vi "TDMSFileViewer KRHPIS_edit - Copy.vi"(4 "error in (no error)":errorcluster, 7 "file path":path) -> (0 "error out":errorcluster, 3 "file path out":path)   [LabVIEW 2015]
doc: "Opens the .tdms file specified in the <B>file path</B> input and presents the file data in the TDMS File Viewer dialog box."
uses:
  <vilib>/Utility/tdmsutil.llb/fileViewerConfigData.ctl
  <vilib>/Utility/error.llb/DialogType.ctl
  <vilib>/Utility/tdmsutil.llb/TDMSFileViewerLocalizedText.vi
  Instance           1 26Saved   TDMS - File Viewer .vi
  <vilib>/Utility/file.llb/Read From Spreadsheet File (DBL).vi
  <vilib>/Analysis/NI_AALPro.lvlib
  <vilib>/Analysis/NI_AALBase.lvlib
panel:
  in  "Help":bool
  in  "Settings...":bool
  in  "Quit":bool
  in  "Status":string
  in  "Properties / Values / Graph":T1(tab)
  in  "Properties":i32(listbox)
  in  "Raw data values":i32(listbox)
  out "Time Difference 2":dbl format="%#_6p"
  out "Amplitude Difference 2":dbl format="%#_6p"
  out "Histogram":T2(graph)
  out "Waveform Graph":waveform(dbl)[](graph)
  out "St. Deviation Qin_1":dbl format="%#.4p"
  out "Variance Qin_1":dbl format="%#.4p"
  out "Mean Qin_1":dbl format="%#.4p"
  out "Mean Qin_2":dbl format="%#.4p"
  out "St. Deviation Qin_2":dbl format="%#.4p"
  out "Variance Qin_2":dbl format="%#.4p"
  out "Gain (mV/fCb)":dbl
  out "Linearity Graph":cluster{"Best Linear Fit":dbl[], "Y":dbl[]}[](graph)
  out "Pulser Waveform":waveform(dbl)[](graph)
  out "Qin 1 (fCb)":dbl format="%#.4p"
  out "Qin 2 (fCb)":dbl format="%#.4p"
  out "Simul. Graph":cluster{"all rows":dbl[], "all rows":dbl[]}[](graph)
  in  "Load simulation Plot":bool
  in  "Cursor.Visible":bool
  in  "Cursor.Visible 2":bool
  out "Time Difference":dbl format="%#_6p"
  out "Amplitude Difference":dbl format="%#_6p"
  in  "File contents":string(tree)
  # "Displaying values 1..1000"
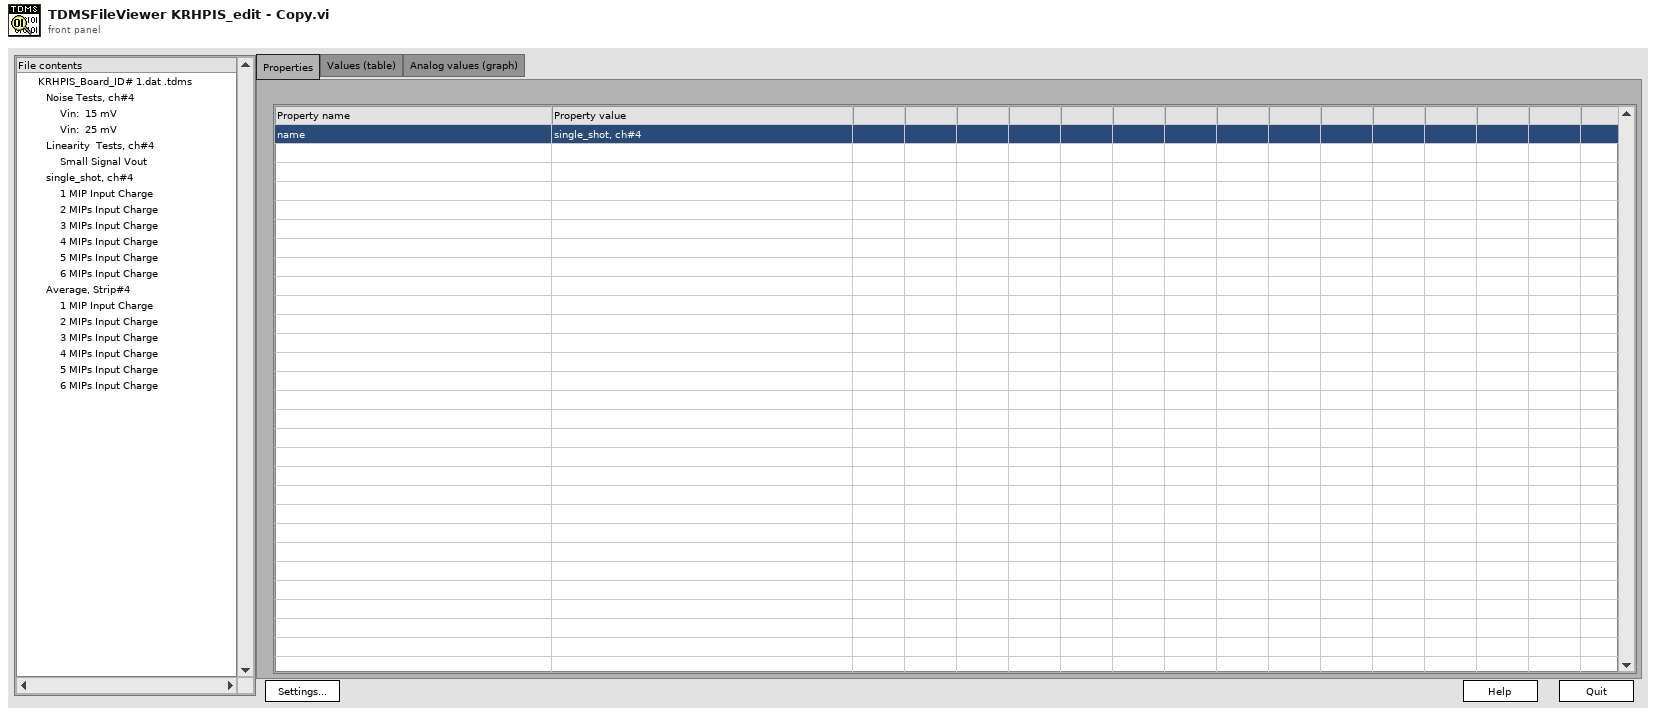
[diagram p1: front panel]
types:
  T1 = enum32{"Properties", "Values (table)", "Analog values (graph)"}
  T2 = cluster{"X Values":dbl[], "Histogram: h(x)":i32[]}[]
  T3 = enum16{"open", "open or create", "create or replace", "create", "open (read-only)"}
  T4 = typedef "fileViewerConfigData.ctl" = cluster{"Show all (table)":bool, "Show all (graph)":bool, "limit (table)":u64, "limit (graph)":u64, "no show":bool, "start (table)":u64, "start (graph)":u64}
  T5 = cluster{"Tree":refnum<vi>, "Tab Control":refnum<vi>, "property list":refnum<vi>, "raw data list":refnum<vi>, "Waveform Graph":refnum<vi>, "Ok":refnum<vi>, "Ok 2":refnum<vi>, "Ok 3":refnum<vi>, "Ok 4":refnum<vi>}
  T6 = cluster{"X Values":dbl[], "Histogram: h(x)":i32[]}
  T7 = typedef "DialogType.ctl" = u16
  T8 = typedef "LVRectTypeDef.ctl" = cluster{"Left":i16, "Top":i16, "Right":i16, "Bottom":i16}
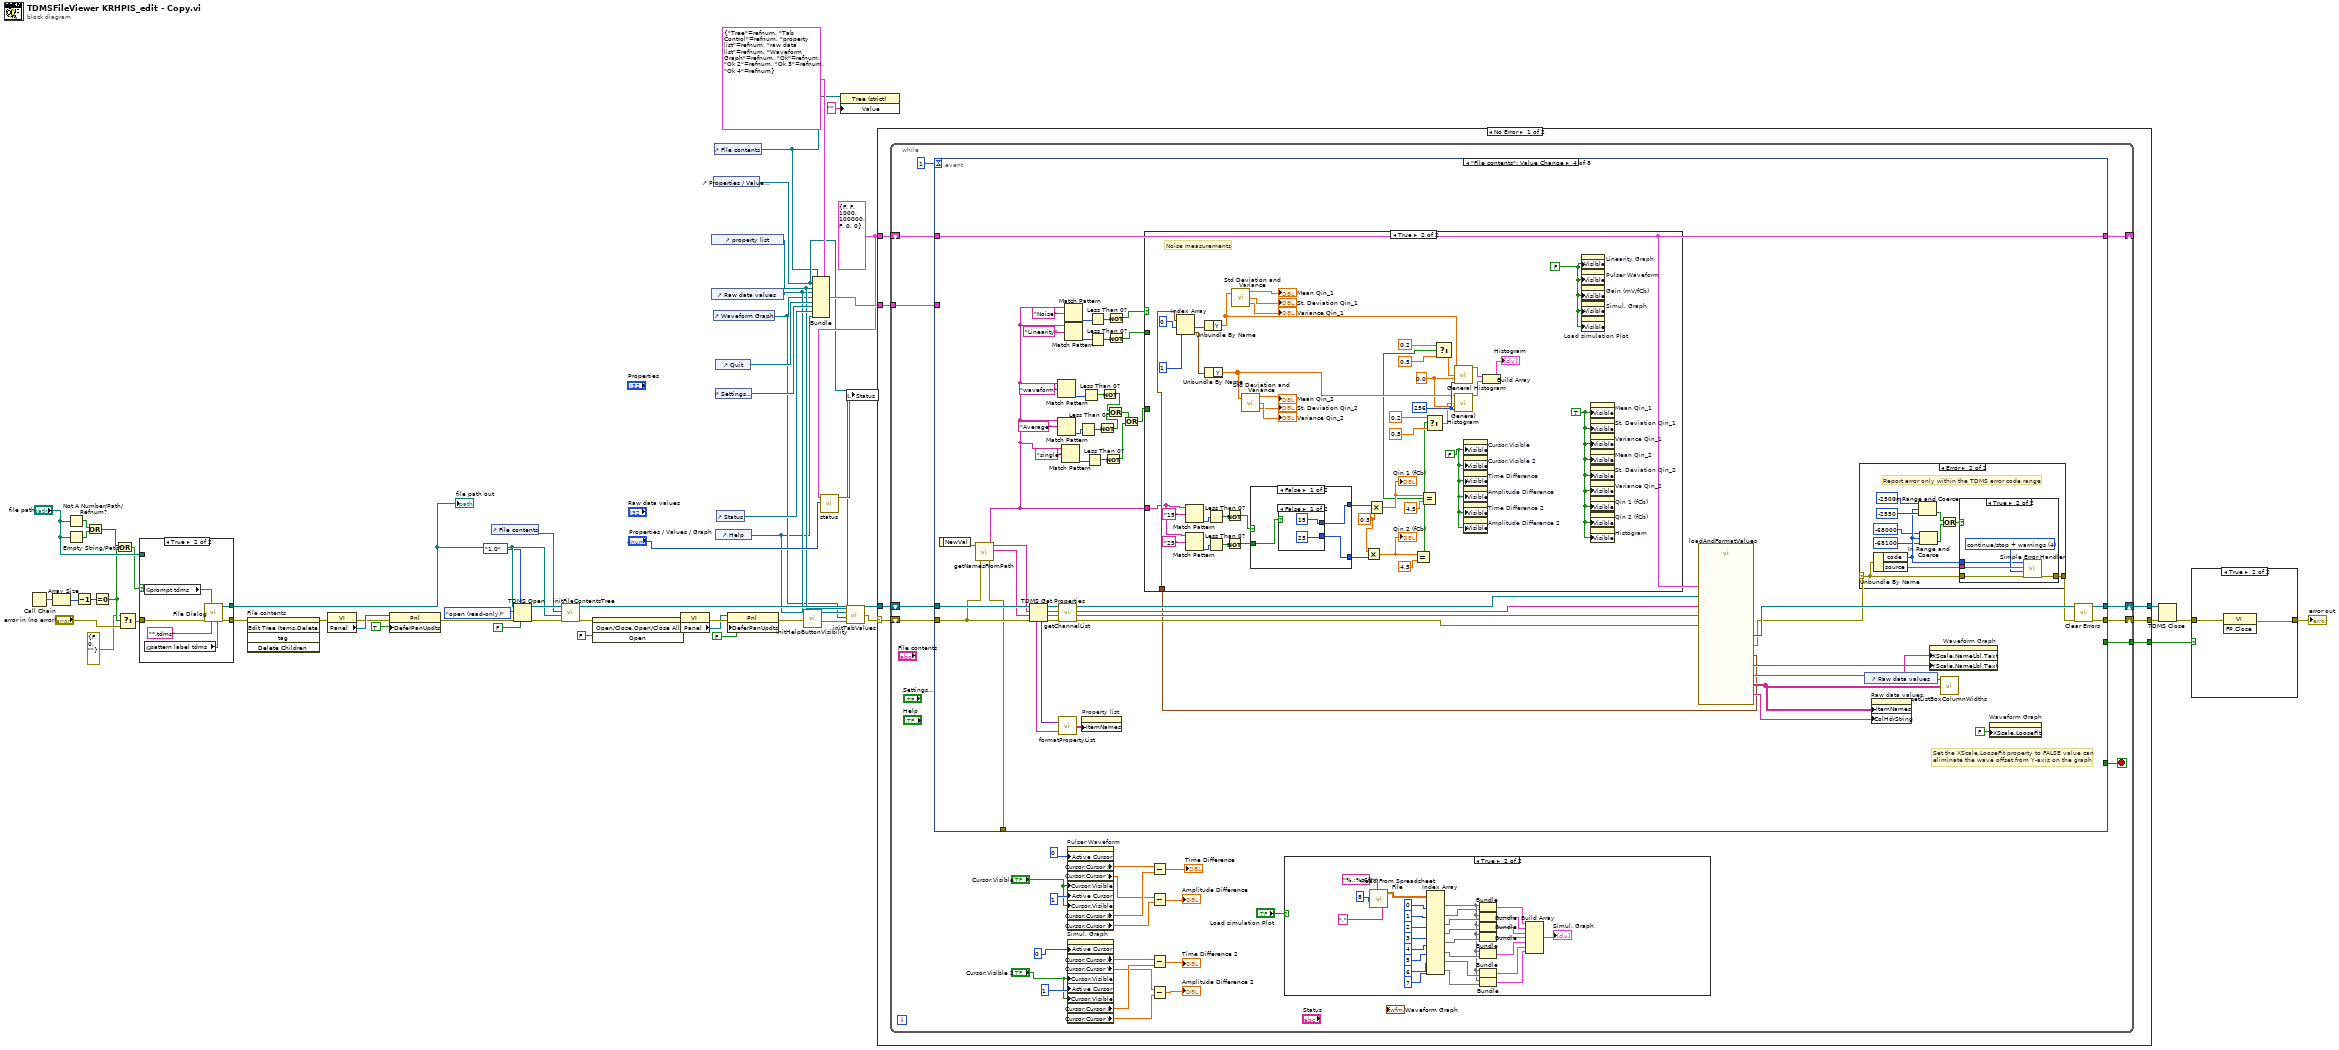
[diagram p0: block diagram]
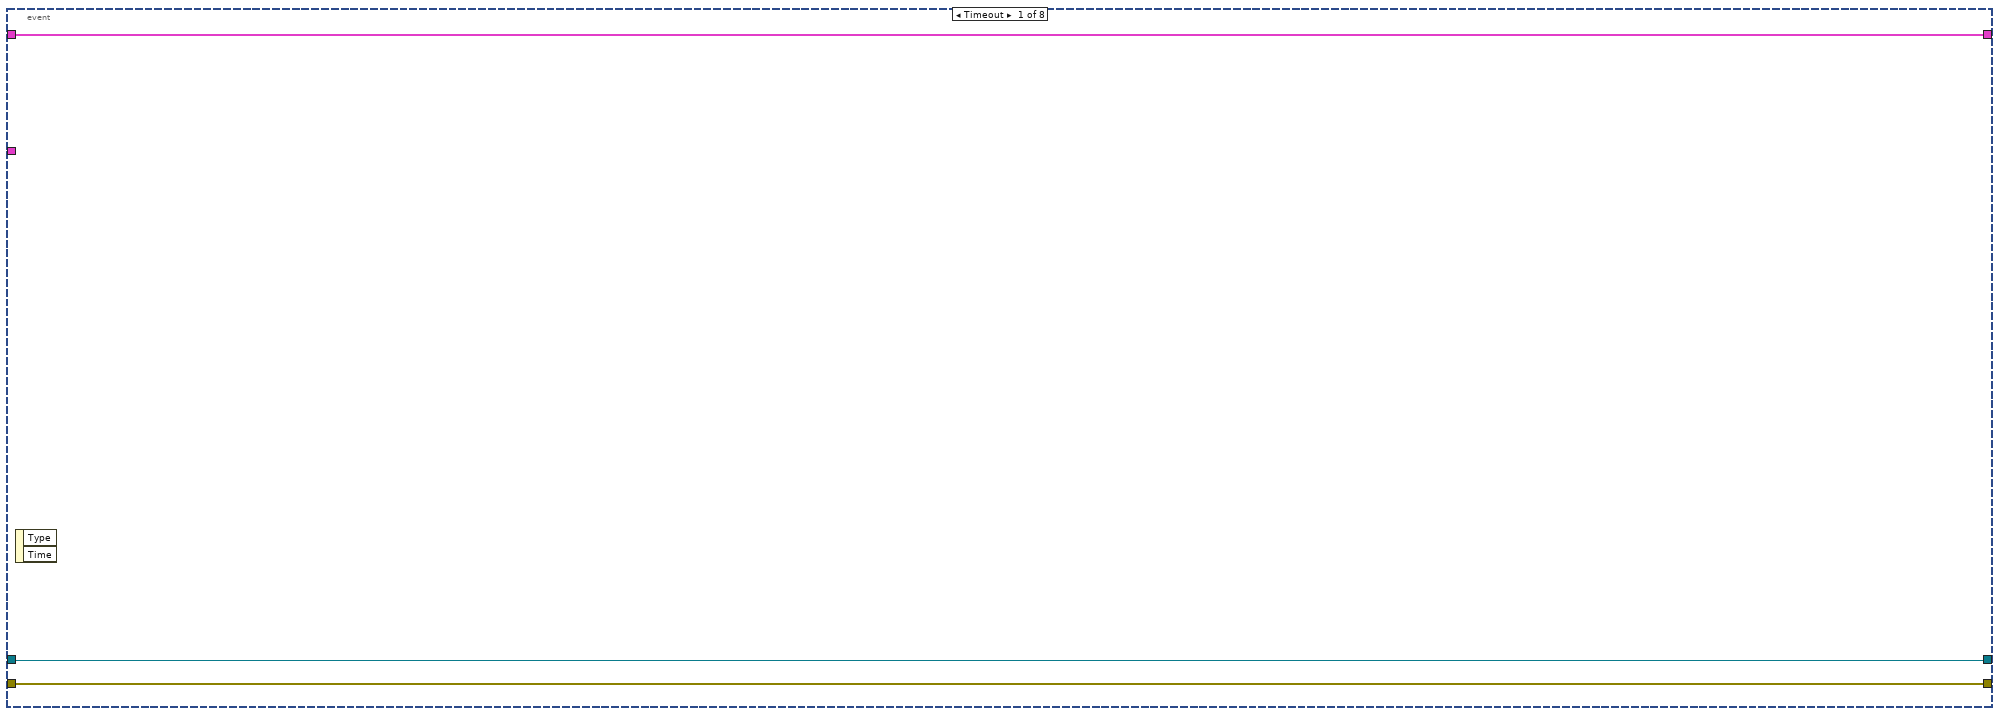
[diagram p4: hidden frame]
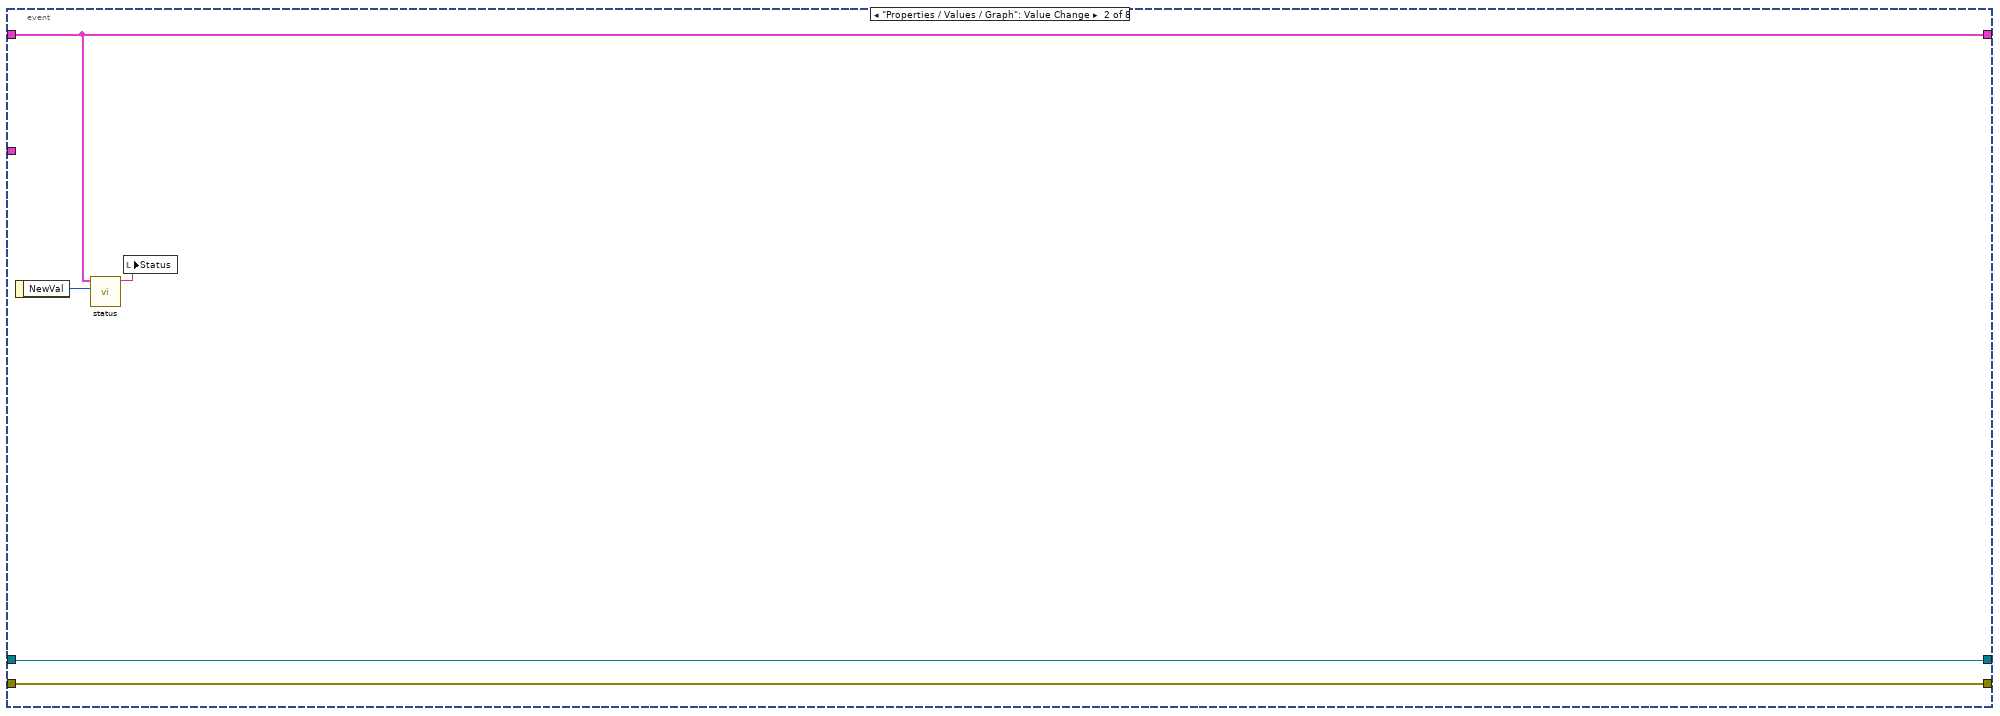
[diagram p5: hidden frame]
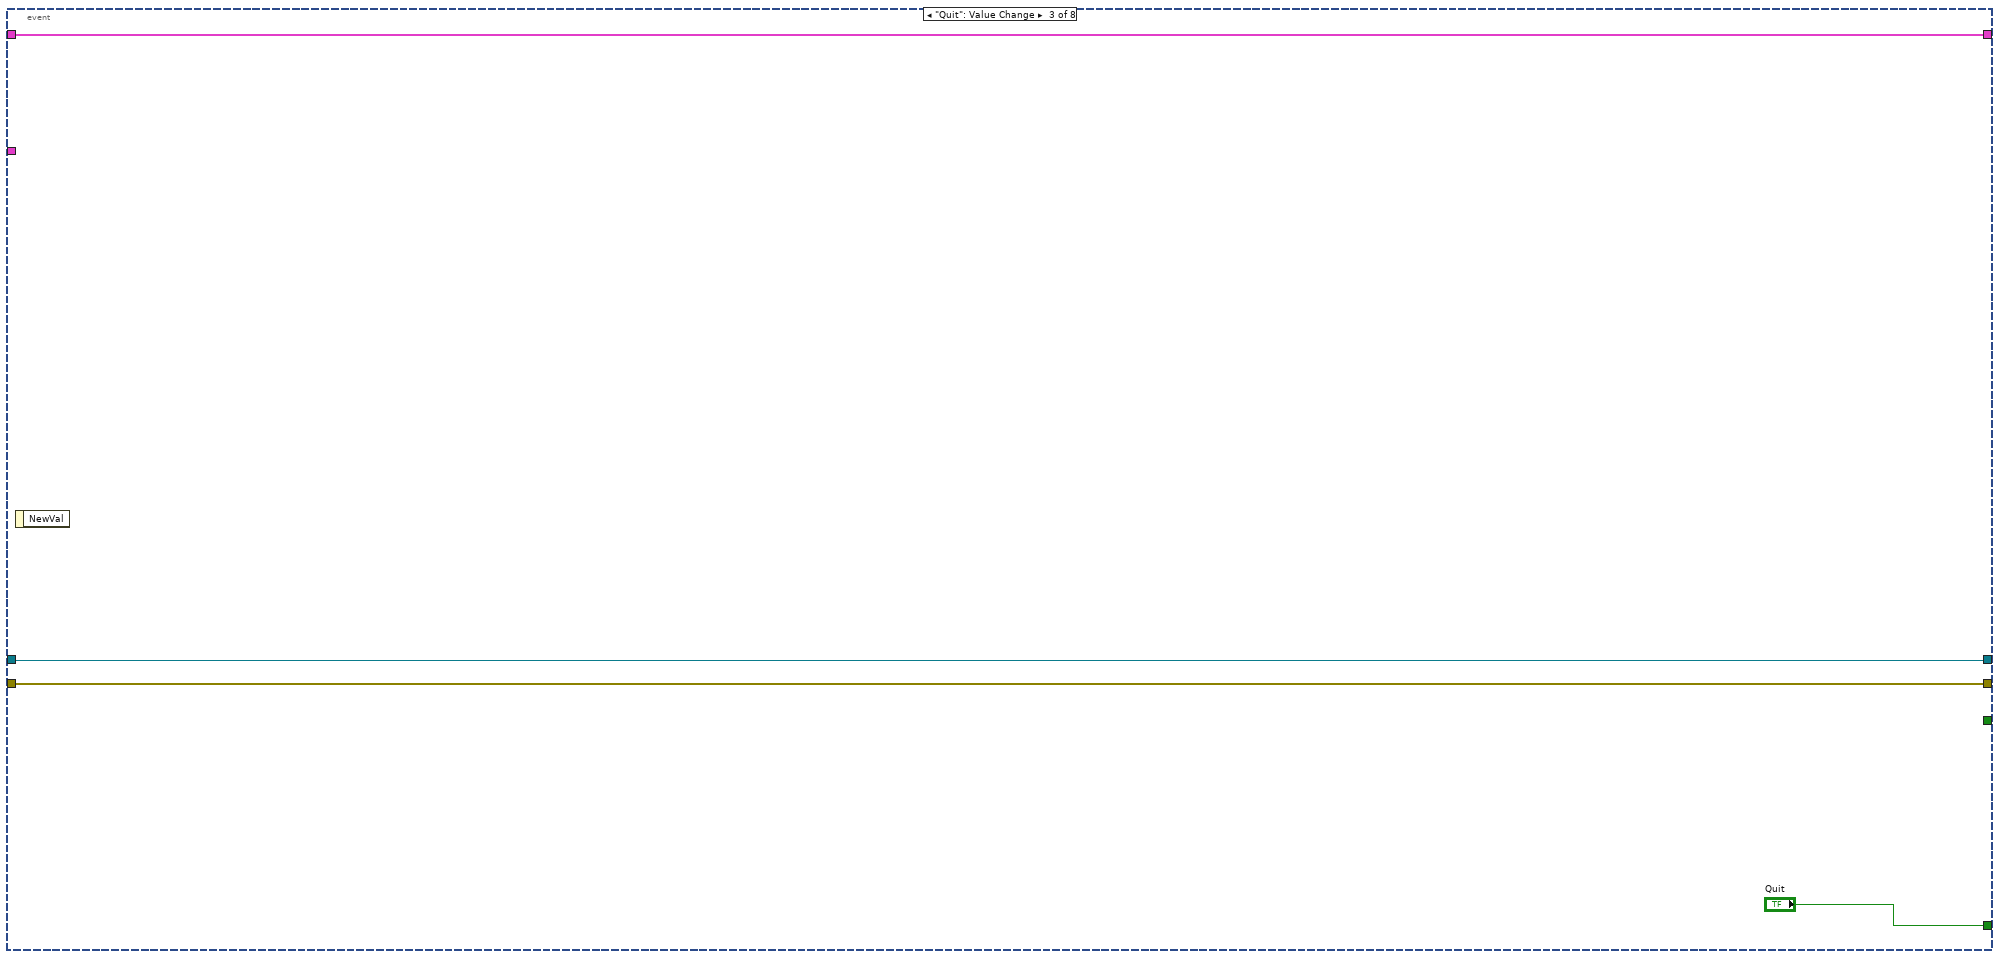
[diagram p6: hidden frame]
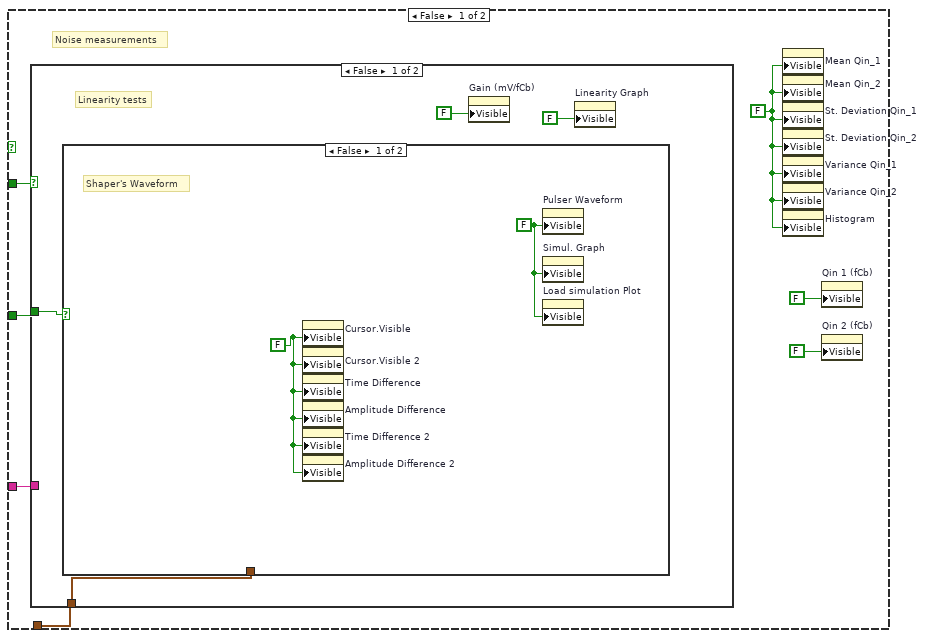
[diagram p7: hidden frame]
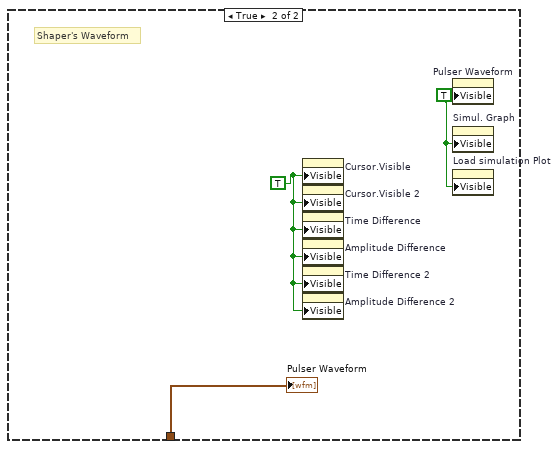
[diagram p8: hidden frame]
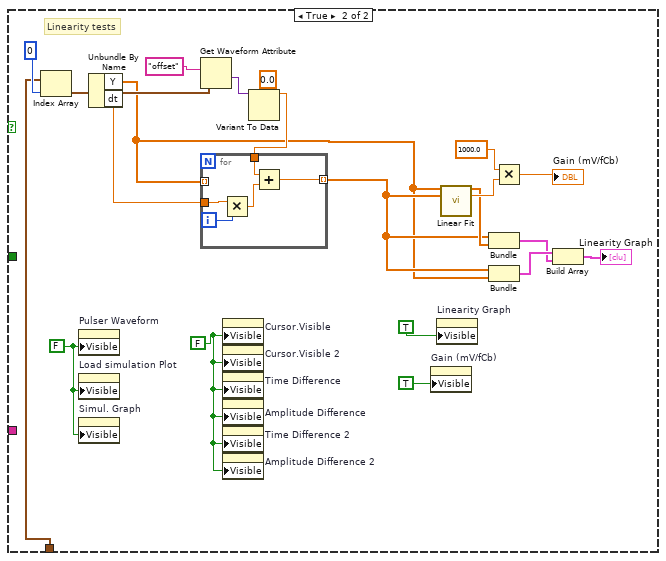
[diagram p9: hidden frame]
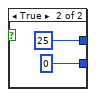
[diagram p10: hidden frame]
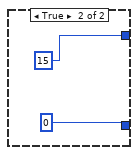
[diagram p11: hidden frame]
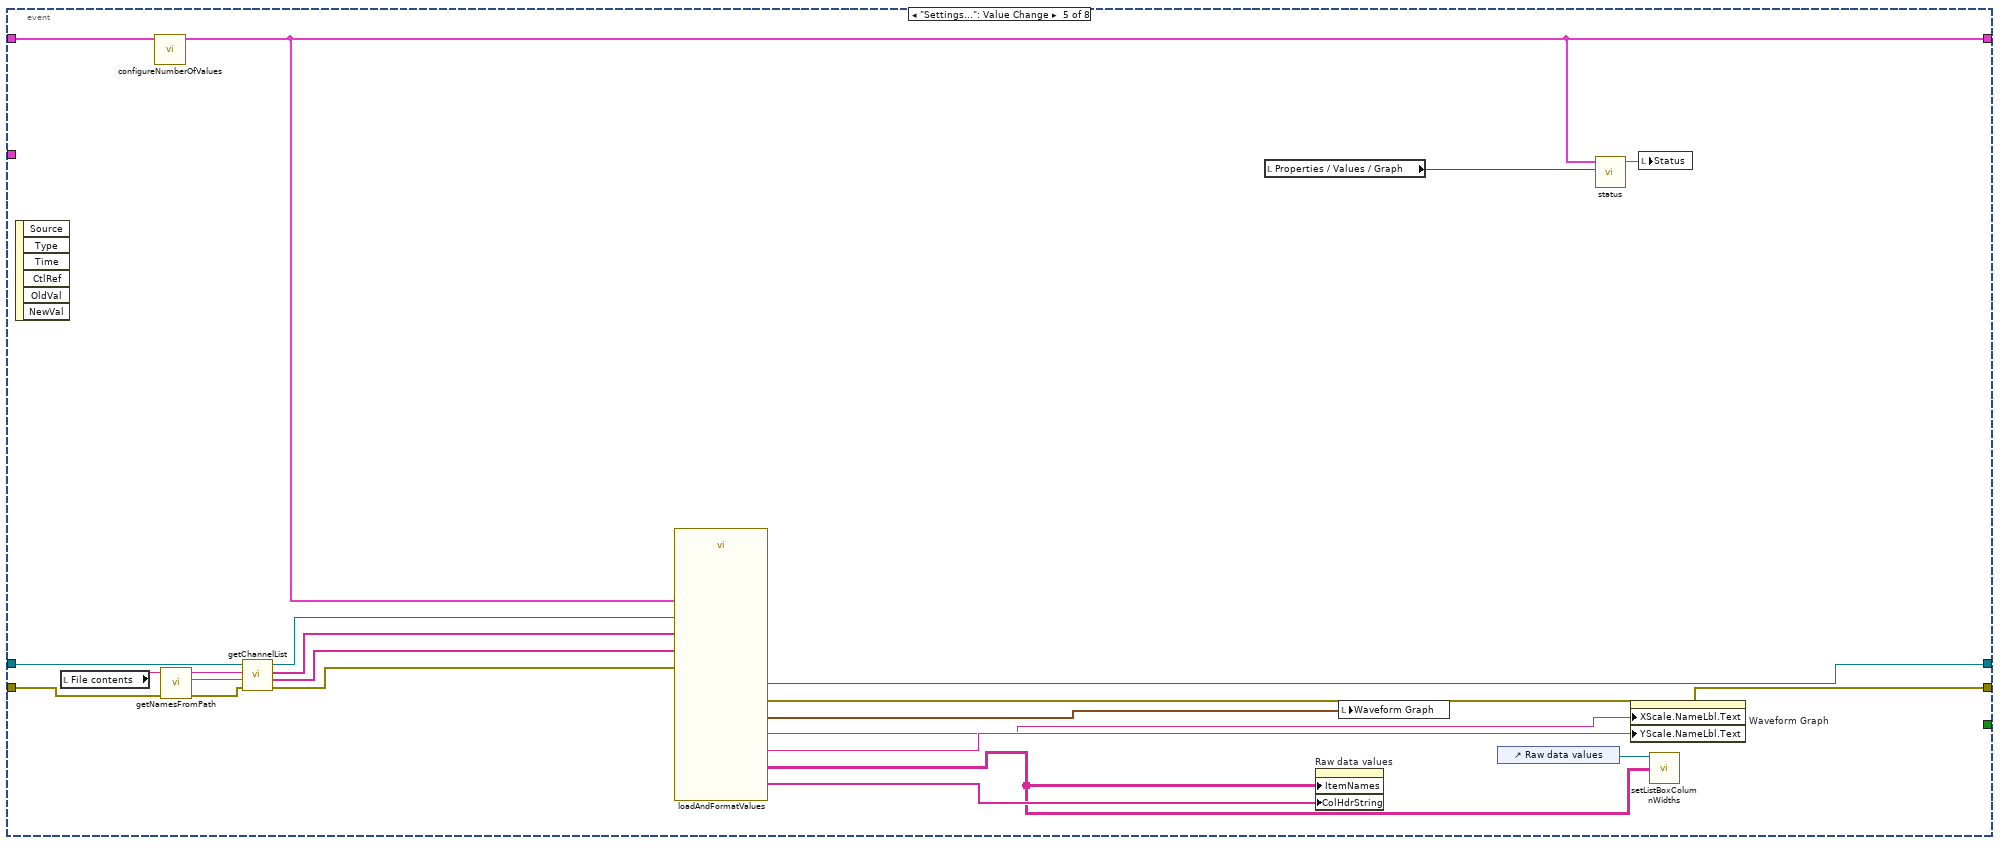
[diagram p14: hidden frame]
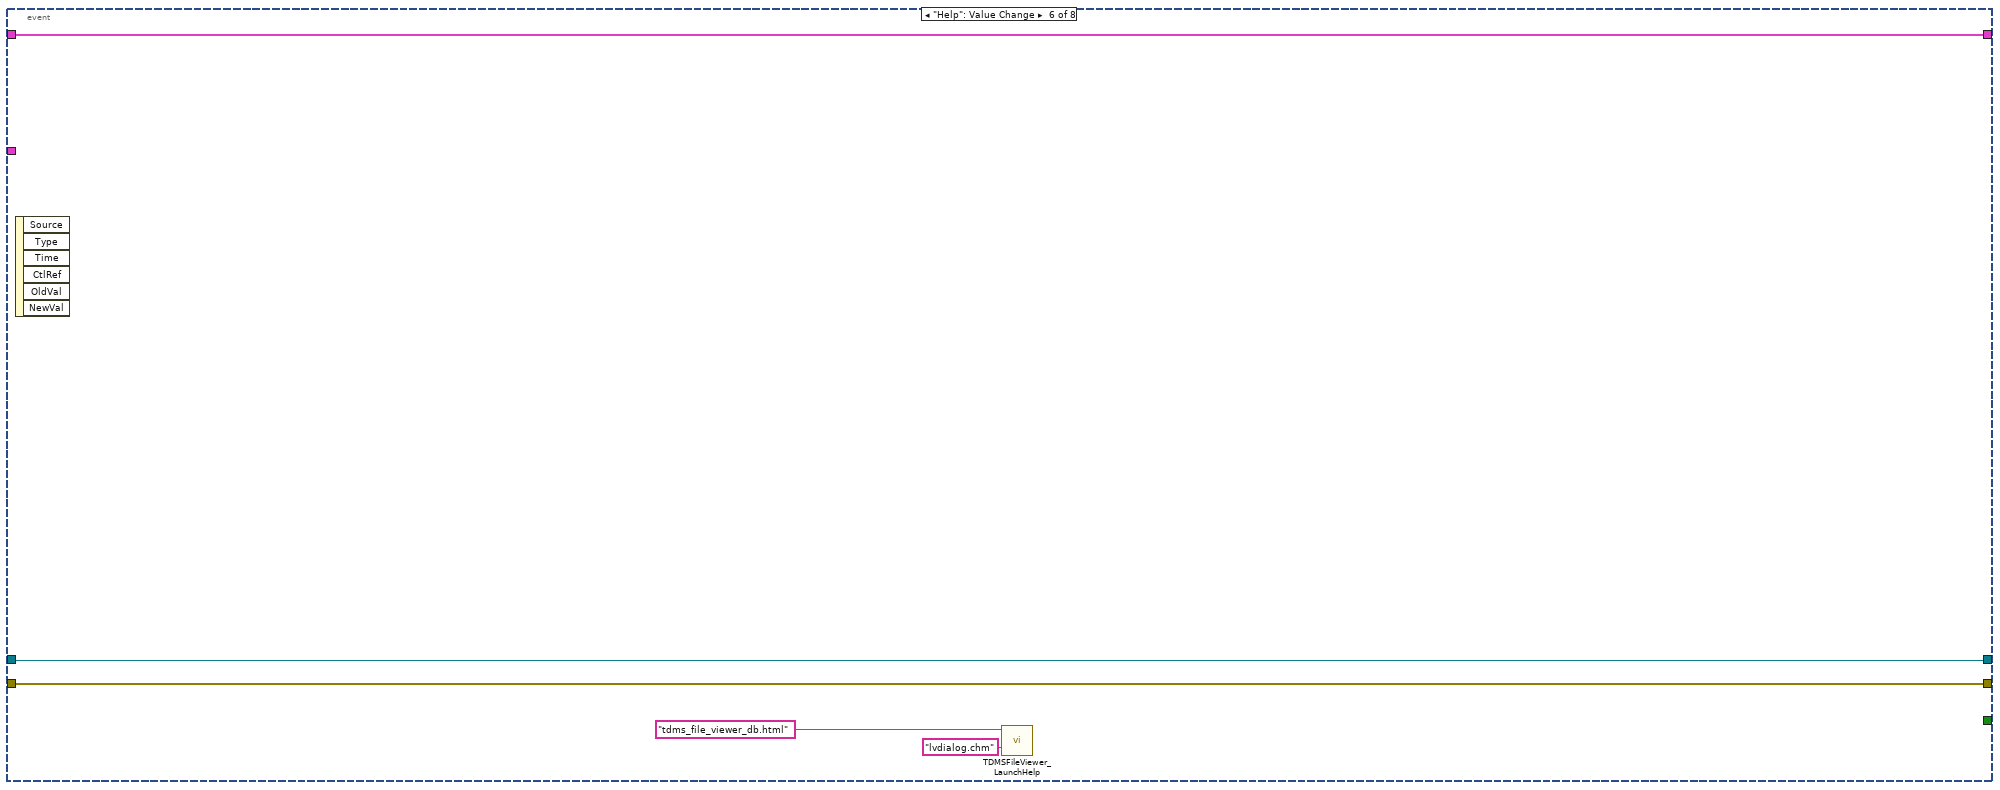
[diagram p15: hidden frame]
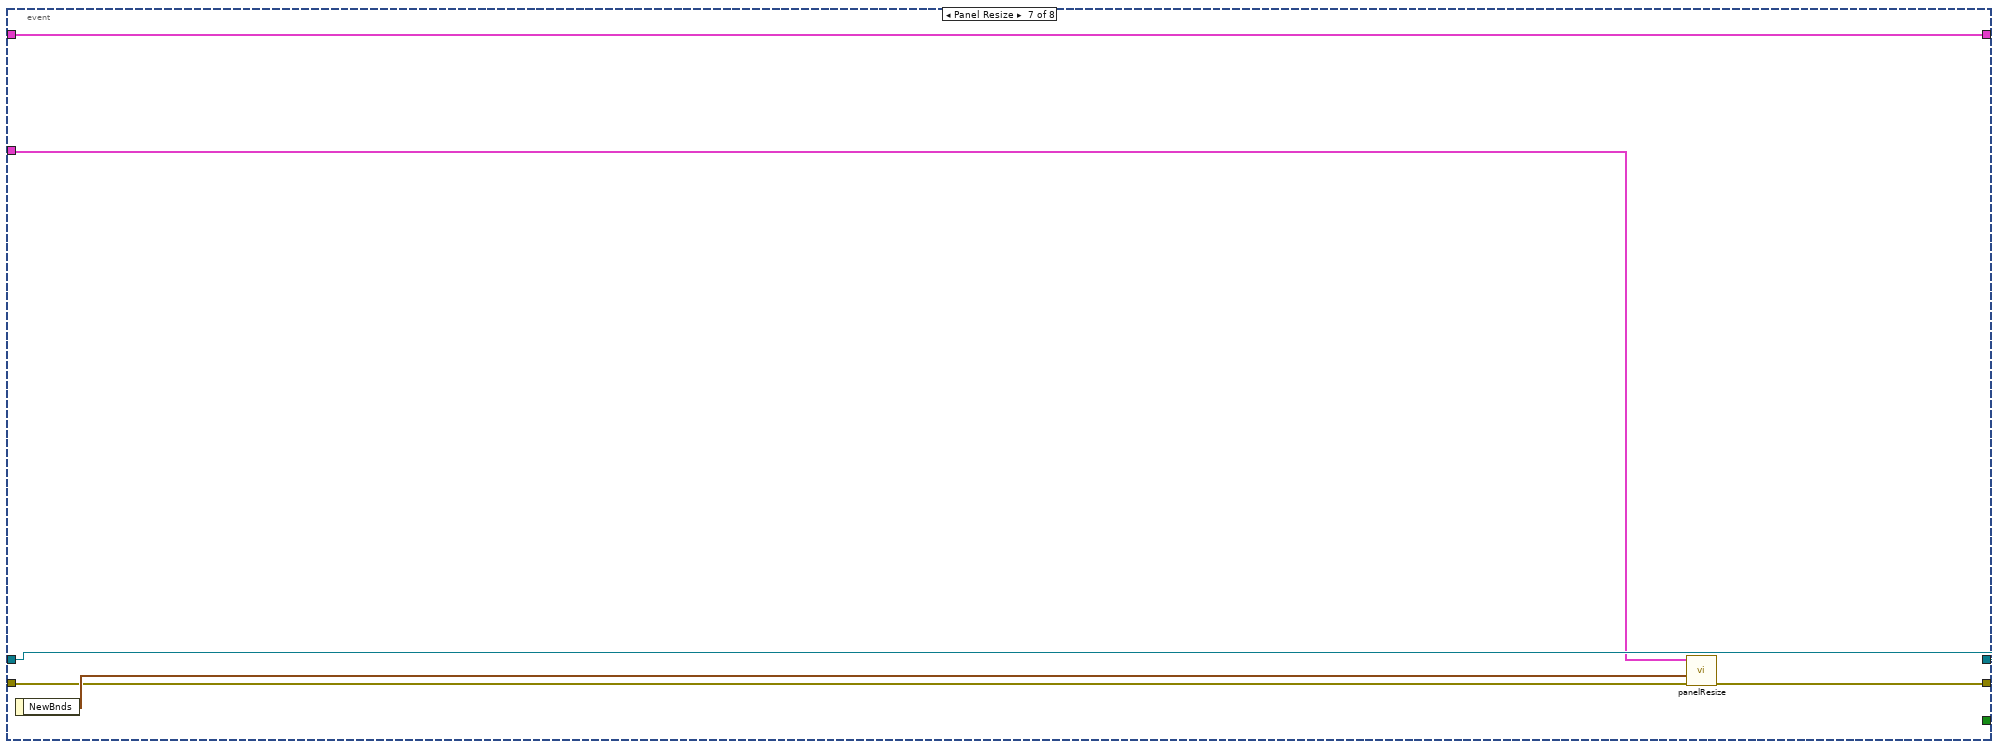
[diagram p16: hidden frame]
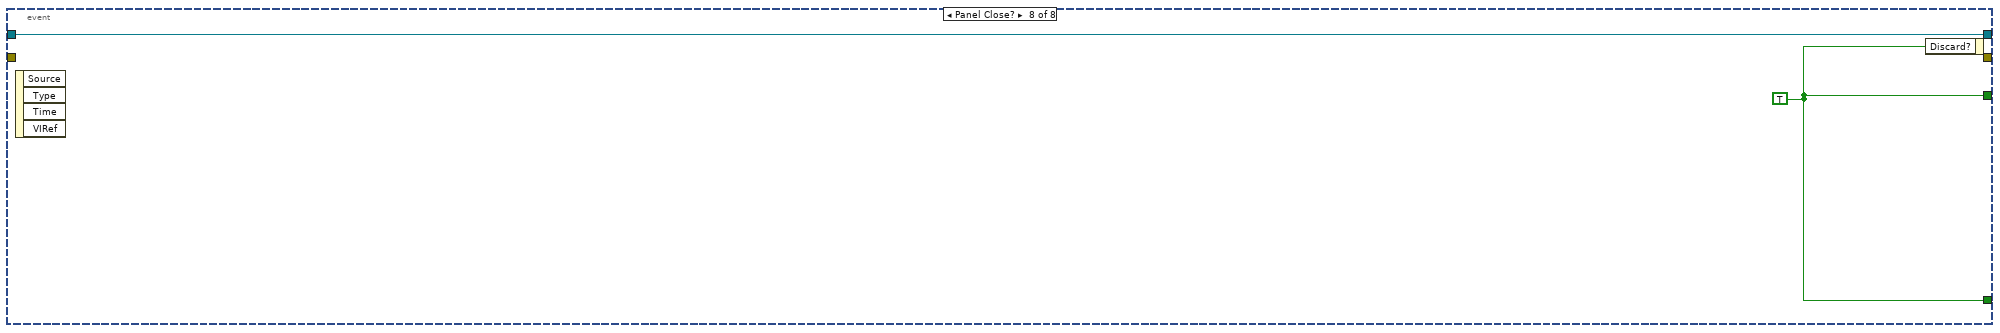
[diagram p17: hidden frame]
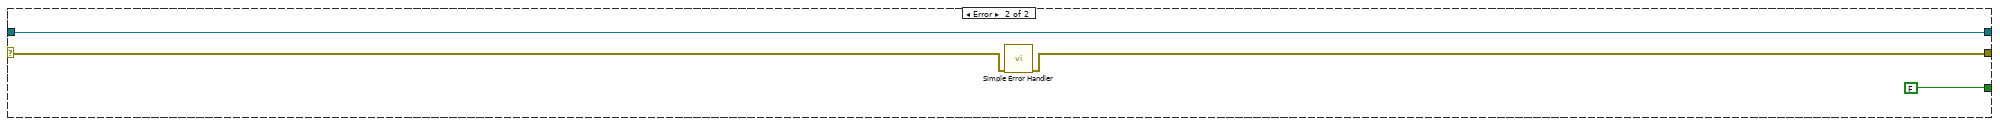
[diagram p18: hidden frame]
diagram:
  w21 = T4 {"Show all (table)"=FALSE, "Show all (graph)"=FALSE, "limit (table)"=1000, "limit (graph)"=100000, "no show"=FALSE, "start (table)"=0, "start (graph)"=0} ("TDMS File Viewer Configuration")
  n1 = Call Chain() -> (call chain=w36:string[])
  n2 = Array Size(array=w36) -> (size(s)=w34:i32)
  n3 = Not A Number/Path/Refnum?(number/path/refnum="file path") -> (NaN/Path/Refnum?=w38:bool)
  n4 = Empty String/Path?(string/path="file path") -> (empty?=w37:bool)
  n5 = Decrement(x=w34) -> (x-1=w33:i32)
  n6 = Or(x=w38, y=w37) -> (x .or. y?=w35:bool)
  n7 = Equal To 0?(x=w33) -> (x = 0?=w19:bool)
  n8 = Or(x=w35, y=w19) -> (x .or. y?=w32:bool)
  n9 = Select(t=errorcluster {"status"=FALSE, "code"=0, "source"=""}, s=w19, f="error in (no error)") -> (s? t:f=w18:errorcluster)
  n10 = case shown="True" w32 {
    tunnel: [w57 w63] -> w25
    tunnel: "file path" -> [w57 _]
    tunnel: [w56 w61] -> w24
    tunnel: w18 -> [w56 w60]
    frame False {
    }
    frame True {
      n11 = global read "TDMSFileViewerLocalizedText.vi" "prompt tdms"() -> (w59:string)
      n12 = global read "TDMSFileViewerLocalizedText.vi" "pattern label tdms"() -> (w58:string)
      n13 = call "File Dialog"("prompt"=w59, "error in"=w60, "pattern (all files)"="*.tdms", "pattern label"=w58) -> ("selected path"=w63:path, "error out"=w61:errorcluster)  [unwired: 3 in, 7 out]
    }
  }
  "file path out" <- w25
  n14 = invoke on="File contents" class="Tree (strict)" method="Edit Tree Items.Delete"(error in=w24) -> (error out=w46:errorcluster)  [unwired: 4 in, 4 out]
  n15 = property class="VI"(error in=w46) -> (error out=w47:errorcluster, "Panel"=w48:refnum<vi>)  [unwired: 1 in, 1 out]
  n16 = property class="Pnl"(reference=w48, error in=w47, "DeferPanUpdts"=TRUE ("Defer Panel Updates")) -> (error out=w50:errorcluster)  [unwired: 1 out]
  n17 = control-ref of="File contents"() -> (w26:refnum<vi>)
  n18 = TDMS Open(6:FALSE ("disable buffering (T)"), 7:enum16{"1.0", "2.0"}."1.0" ("file format version (2.0)"), 8:w50, 10:T3."open (read-only)" ("operation"), 11:w25) -> (0:w55:errorcluster, 3:w54:refnum<k34>)  [unwired: 2 in]
  n19 = call <vilib>:"initFileContentsTree.vi"("error in (no error)"=w55, "file path"=w25, "Tree Refnum"=w26, "tdms file"=w54) -> ("error out"=w42:errorcluster, "tdms file out"=w53:refnum<k34>)  [unwired: 2 out]
  n20 = invoke on="File contents" class="Tree (strict)" method="Open/Close.Open/Close All"(error in=w42, "Open"=FALSE ("Open?")) -> (error out=w41:errorcluster)  [unwired: 2 in, 3 out]
  n21 = property class="VI"(error in=w41) -> (error out=w44:errorcluster, "Panel"=w43:refnum<vi>)  [unwired: 1 in, 1 out]
  n22 = control-ref of="property list"() -> (w9:refnum<vi>)
  n23 = control-ref of="Raw data values"() -> (w8:refnum<vi>)
  n24 = control-ref of="Properties / Values / Graph"() -> (w6:refnum<vi>)
  n25 = control-ref of="Waveform Graph"() -> (w7:refnum<vi>)
  n26 = control-ref of="File contents"() -> (w5:refnum<vi>)
  n27 = control-ref of="Quit"() -> (w30:refnum<vi>)
  n28 = control-ref of="Settings..."() -> (w28:refnum<vi>)
  n29 = control-ref of="Help"() -> (w1:refnum<vi>)
  n30 = control-ref of="Status"() -> (w23:refnum<vi>)
  n31 = property class="Pnl"(reference=w43, error in=w44, "DeferPanUpdts"=FALSE ("Defer Panel Updates")) -> (error out=w3:errorcluster)  [unwired: 1 out]
  n32 = call <vilib>:"initHelpButtonVisibility.vi"("error in"=w3, "Help"=w1) -> ("error out"=w2:errorcluster)  [unwired: 9 in]
  n33 = Bundle(cluster=T5 {"Tree"=refnum, "Tab Control"=refnum, "property list"=refnum, "raw data list"=refnum, "Waveform Graph"=refnum, "Ok"=refnum, "Ok 2"=refnum, "Ok 3"=refnum, "Ok 4"=refnum} ("control refs"), "Tree"=w5, "Tab Control"=w6, "property list"=w9, "raw data list"=w8, "Waveform Graph"=w7, "Ok"=w30, "Ok 2"=w28, "Ok 3"=w23, "Ok 4"=w1) -> (w31:T5)
  n34 = call <vilib>:"status.vi"("tab sheet"="Properties / Values / Graph", "TDMS File Viewer Configuration"=w21) -> ("status"=w22:string)  [unwired: 5 out]
  n35 = property class="Tree (strict)"(reference=w5, "Value"="") -> ()  [unwired: 1 in, 2 out]
  n36 = local write "Status"(w22) -> ()
  n37 = call <vilib>:"initTabValues.vi"("properties"=w9, "Values"=w8, "waveform"=w7, "error in"=w2, "Properties / Values / Graph"=w6) -> ("error out"=w10:errorcluster)
  n38 = case shown="No Error" w10 {
    selector: w10 -> [w65 w342]
    tunnel: w53 -> [w70 w343]
    tunnel: [w69 w343] -> w52
    tunnel: [w68 w341] -> w51
    tunnel: w31 -> [w67 _]
    tunnel: w21 -> [w66 _]
    tunnel: [w64 FALSE] -> w15
    frame No Error {
      n39 = while {
        shift-right: [w97] -> w68
        shift-left: w65 -> [w98]
        shift-right: [w96] -> w69
        shift-left: w70 -> [w99]
        tunnel: w67 -> [w94]
        shift-right: [w92] -> _
        shift-left: w66 -> [w93]
        tunnel: [w91] -> w64
        stop <- w95 stop-if-true
        n40 = event shown="[3] \"File contents\": Value Change" {
          selector: _ -> [_ _ _ _ _ _ _ _]
          dyn-events: _ -> [_ _ _ _ _ _ _ _]
          timeout: 1 -> [_ _ _ _ _ _ _ _]
          tunnel: w99 -> [w129 w134 w138 w190 w315 w330 w337 w339]
          tunnel: w98 -> [w130 w135 w137 w183 w323 w329 w334 _]
          tunnel: [w130 w135 w137 w179 w324 w329 w333 _] -> w97
          tunnel: [w129 w134 w138 w189 w325 w330 w337 w339] -> w96
          tunnel: [_ _ "Quit" _ _ _ _ w338] -> w95
          tunnel: [_ _ _ w182 _ _ _ _] -> _
          tunnel: w94 -> [_ _ _ _ _ _ w335 _]
          tunnel: w93 -> [w128 w131 w136 w172 w326 w331 w332 _]
          tunnel: [w128 w131 w136 w172 w305 w331 w332 _] -> w92
          tunnel: [_ _ _ _ _ _ _ w338] -> w91
          event Timeout {
            n41 = event-data() -> ()  [unwired: 3 out]
          }
          event "Properties / Values / Graph": Value Change {
            n42 = event-data() -> ("NewVal"=w133:T1)  [unwired: 1 out]
            n43 = call <vilib>:"status.vi"("tab sheet"=w133, "TDMS File Viewer Configuration"=w131) -> ("status"=w132:string)  [unwired: 5 out]
            n44 = local write "Status"(w132) -> ()
          }
          event "Quit": Value Change {
            n45 = event-data() -> ()  [unwired: 2 out]
          }
          event "File contents": Value Change {
            # "Set the XScale.LooseFit property to FALSE value can \neliminate the wave offset from Y-axis on the graph"
            n46 = event-data() -> ("NewVal"=w143:string)  [unwired: 1 out]
            n47 = call <vilib>:"getNamesFromPath.vi"("error in (no error)"=w183, "tree path"=w143) -> ("error out"=w182:errorcluster, "channel"=w187:string, "group"=w188:string)  [unwired: 3 out]
            n48 = TDMS Get Properties(8:w183, 9:w187, 10:w188, 11:w190) -> (0:w177:errorcluster, 1:w176:string, 2:w171:string, 3:w178:refnum<k34>, 4:w185:variant[], 6:w186:string[])  [unwired: 2 out]
            n49 = Match Pattern(string=w143, regular expression="waveform") -> (offset past match=w158:i32)  [unwired: 1 in, 3 out]
            n50 = Match Pattern(string=w143, regular expression="Average") -> (offset past match=w150:i32)  [unwired: 1 in, 3 out]
            n51 = call <vilib>:"getChannelList.vi"("error in (no error)"=w177, "channel names"=w176, "group name"=w171, "tdms file"=w178) -> ("error out"=w167:errorcluster, "channel names out"=w168:string[], "group names out"=w169:string[], "tdms file out"=w170:refnum<k34>)
            n52 = call <vilib>:"formatPropertyList.vi"("property names"=w186, "property values"=w185) -> ("strings"=w184:string[][])
            n53 = Match Pattern(string=w143, regular expression="single") -> (offset past match=w145:i32)  [unwired: 1 in, 3 out]
            n54 = Match Pattern(string=w143, regular expression="Noise") -> (offset past match=w162:i32)  [unwired: 1 in, 3 out]
            n55 = Match Pattern(string=w143, regular expression="Linearity") -> (offset past match=w160:i32)  [unwired: 1 in, 3 out]
            n56 = Less Than 0?(x=w150) -> (x < 0?=w151:bool)
            n57 = property on="Property list" class="MCListbox (strict)"("ItemNames"=w184) -> ()  [unwired: 2 in, 2 out]
            n58 = Less Than 0?(x=w158) -> (x < 0?=w155:bool)
            n59 = Less Than 0?(x=w145) -> (x < 0?=w144:bool)
            n60 = Less Than 0?(x=w162) -> (x < 0?=w157:bool)
            n61 = Less Than 0?(x=w160) -> (x < 0?=w156:bool)
            n62 = Not(x=w151) -> (.not. x?=w149:bool)
            n63 = Not(x=w155) -> (.not. x?=w148:bool)
            n64 = Not(x=w144) -> (.not. x?=w142:bool)
            n65 = Or(x=w148, y=w149) -> (x .or. y?=w141:bool)
            n66 = Not(x=w157) -> (.not. x?=w154:bool)
            n67 = Not(x=w156) -> (.not. x?=w153:bool)
            n68 = Or(x=w141, y=w142) -> (x .or. y?=w140:bool)
            n69 = call <vilib>:"loadAndFormatValues.vi"("error in (no error)"=w167, "configuration"=w172, "channel names"=w168, "group names"=w169, "tdms file"=w170) -> ("error out"=w166:errorcluster, "graph y names"=w174:string, "graph x names"=w173:string, "tdms file out"=w189:refnum<k34>, "waveform values"=w147:waveform(dbl)[], "table values"=w181:string[][], "table headers"=w175:string[])
            n70 = case shown="True" w154 {
              tunnel: w147 -> [w196 w267]
              tunnel: w153 -> [w197 _]
              tunnel: w143 -> [w195 w253]
              tunnel: w140 -> [w194 _]
              frame False {
                w193 = FALSE ("Visible")
                # "Noise measurements"
                n71 = case shown="False" w197 {
                  tunnel: w196 -> [w199 w226]
                  tunnel: w195 -> [_ _]
                  tunnel: w194 -> [w201 _]
                  frame False {
                    # "Linearity tests"
                    n72 = case shown="False" w201 {
                      tunnel: w199 -> [_ w206]
                      frame False {
                        w202 = FALSE ("Cursor.Visible")
                        w203 = FALSE ("Visible")
                        # "Shaper's Waveform"
                        n73 = property on="Cursor.Visible" class="Bool (strict)"("Visible"=w202) -> ()  [unwired: 2 in, 2 out]
                        n74 = property on="Cursor.Visible 2" class="Bool (strict)"("Visible"=w202) -> ()  [unwired: 2 in, 2 out]
                        n75 = property on="Time Difference" class="DigNum (strict)"("Visible"=w202) -> ()  [unwired: 2 in, 2 out]
                        n76 = property on="Amplitude Difference" class="DigNum (strict)"("Visible"=w202) -> ()  [unwired: 2 in, 2 out]
                        n77 = property on="Time Difference 2" class="DigNum (strict)"("Visible"=w202) -> ()  [unwired: 2 in, 2 out]
                        n78 = property on="Amplitude Difference 2" class="DigNum (strict)"("Visible"=w202) -> ()  [unwired: 2 in, 2 out]
                        n79 = property on="Pulser Waveform" class="WFGraph (strict)"("Visible"=w203) -> ()  [unwired: 2 in, 2 out]
                        n80 = property on="Simul. Graph" class="XYGraph (strict)"("Visible"=w203) -> ()  [unwired: 2 in, 2 out]
                        n81 = property on="Load simulation Plot" class="Bool"("Visible"=w203) -> ()  [unwired: 2 in, 2 out]
                      }
                      frame True {
                        w204 = TRUE ("Cursor.Visible")
                        w205 = TRUE ("Visible")
                        # "Shaper's Waveform"
                        n82 = property on="Cursor.Visible" class="Bool (strict)"("Visible"=w204) -> ()  [unwired: 2 in, 2 out]
                        n83 = property on="Cursor.Visible 2" class="Bool (strict)"("Visible"=w204) -> ()  [unwired: 2 in, 2 out]
                        n84 = property on="Time Difference" class="DigNum (strict)"("Visible"=w204) -> ()  [unwired: 2 in, 2 out]
                        n85 = property on="Amplitude Difference" class="DigNum (strict)"("Visible"=w204) -> ()  [unwired: 2 in, 2 out]
                        n86 = property on="Time Difference 2" class="DigNum (strict)"("Visible"=w204) -> ()  [unwired: 2 in, 2 out]
                        n87 = property on="Amplitude Difference 2" class="DigNum (strict)"("Visible"=w204) -> ()  [unwired: 2 in, 2 out]
                        n88 = property on="Pulser Waveform" class="WFGraph (strict)"("Visible"=w205) -> ()  [unwired: 2 in, 2 out]
                        n89 = property on="Simul. Graph" class="XYGraph (strict)"("Visible"=w205) -> ()  [unwired: 2 in, 2 out]
                        n90 = property on="Load simulation Plot" class="Bool"("Visible"=w205) -> ()  [unwired: 2 in, 2 out]
                        "Pulser Waveform" <- w206
                      }
                    }
                    n91 = property on="Gain (mV/fCb)" class="DigNum (strict)"("Visible"=FALSE) -> ()  [unwired: 2 in, 2 out]
                    n92 = property on="Linearity Graph" class="XYGraph (strict)"("Visible"=FALSE) -> ()  [unwired: 2 in, 2 out]
                  }
                  frame True {
                    w216 = FALSE ("Cursor.Visible")
                    w217 = FALSE ("Visible")
                    # "Linearity tests"
                    n93 = Index Array(array=w226, index=0) -> (element=w214:waveform(dbl))
                    n94 = property on="Pulser Waveform" class="WFGraph (strict)"("Visible"=w217) -> ()  [unwired: 2 in, 2 out]
                    n95 = property on="Load simulation Plot" class="Bool"("Visible"=w217) -> ()  [unwired: 2 in, 2 out]
                    n96 = property on="Simul. Graph" class="XYGraph (strict)"("Visible"=w217) -> ()  [unwired: 2 in, 2 out]
                    n97 = Unbundle By Name(w214) -> ("Y"=w207:dbl[], "dt"=w210:dbl)
                    n98 = Get Waveform Attribute(6:"offset" ("name"), 7:w214) -> (1:w212:variant)  [unwired: 2 in, 3 out]
                    n99 = property on="Cursor.Visible" class="Bool (strict)"("Visible"=w216) -> ()  [unwired: 2 in, 2 out]
                    n100 = property on="Cursor.Visible 2" class="Bool (strict)"("Visible"=w216) -> ()  [unwired: 2 in, 2 out]
                    n101 = property on="Time Difference" class="DigNum (strict)"("Visible"=w216) -> ()  [unwired: 2 in, 2 out]
                    n102 = property on="Amplitude Difference" class="DigNum (strict)"("Visible"=w216) -> ()  [unwired: 2 in, 2 out]
                    n103 = property on="Time Difference 2" class="DigNum (strict)"("Visible"=w216) -> ()  [unwired: 2 in, 2 out]
                    n104 = property on="Amplitude Difference 2" class="DigNum (strict)"("Visible"=w216) -> ()  [unwired: 2 in, 2 out]
                    n105 = Variant To Data(type=0.0, Variant=w212) -> (data=w209:dbl)  [unwired: 1 in, 1 out]
                    n106 = for {
                      tunnel: w207 -> [_] mode=indexing
                      tunnel: w210 -> [w232]
                      tunnel: w209 -> [w229]
                      tunnel: [w228] -> w208 mode=indexing
                      i -> [w231]
                      n107 = Multiply(x=w232, y=w231) -> (x*y=w230:dbl)
                      n108 = Add(x=w229, y=w230) -> (x+y=w228:dbl)
                    }
                    n109 = property on="Gain (mV/fCb)" class="DigNum (strict)"("Visible"=TRUE) -> ()  [unwired: 2 in, 2 out]
                    n110 = property on="Linearity Graph" class="XYGraph (strict)"("Visible"=TRUE) -> ()  [unwired: 2 in, 2 out]
                    n111 = call <vilib>:"Linear Fit.vi"("Y"=w207, "X"=w208) -> ("Best Linear Fit"=w215:dbl[], "slope"=w223:dbl)  [unwired: 9 in, 3 out]
                    n112 = Bundle(w208, "Best Linear Fit"=w215) -> (w224:cluster{dbl[], "Best Linear Fit":dbl[]})  [unwired: 1 in]
                    n113 = Bundle(w208, "Y"=w207) -> (w225:cluster{dbl[], "Y":dbl[]})  [unwired: 1 in]
                    n114 = Multiply(x=1000.0, y=w223) -> (x*y=→"Gain (mV/fCb)":dbl)
                    n115 = Build Array(w225, w224) -> (→"Linearity Graph":cluster{dbl[], "Best Linear Fit":dbl[]}[])
                  }
                }
                n116 = property on="Mean Qin_1" class="DigNum (strict)"("Visible"=w193) -> ()  [unwired: 2 in, 2 out]
                n117 = property on="Mean Qin_2" class="DigNum (strict)"("Visible"=w193) -> ()  [unwired: 2 in, 2 out]
                n118 = property on="St. Deviation Qin_1" class="DigNum (strict)"("Visible"=w193) -> ()  [unwired: 2 in, 2 out]
                n119 = property on="St. Deviation Qin_2" class="DigNum (strict)"("Visible"=w193) -> ()  [unwired: 2 in, 2 out]
                n120 = property on="Variance Qin_1" class="DigNum (strict)"("Visible"=w193) -> ()  [unwired: 2 in, 2 out]
                n121 = property on="Variance Qin_2" class="DigNum (strict)"("Visible"=w193) -> ()  [unwired: 2 in, 2 out]
                n122 = property on="Histogram" class="XYGraph (strict)"("Visible"=w193) -> ()  [unwired: 2 in, 2 out]
                n123 = property on="Qin 1 (fCb)" class="DigNum (strict)"("Visible"=FALSE) -> ()  [unwired: 2 in, 2 out]
                n124 = property on="Qin 2 (fCb)" class="DigNum (strict)"("Visible"=FALSE) -> ()  [unwired: 2 in, 2 out]
              }
              frame True {
                w233 = FALSE ("Cursor.Visible")
                w250 = 0.3 ("y")
                w235 = FALSE ("Visible")
                w234 = TRUE ("Visible")
                w248 = 0.0 ("min")
                w264 = 256 ("# bins")
                # "Noise measurements"
                n125 = Index Array(array=w267, index #1=0 ("index"), index #2=1 ("index")) -> (element #1=w268:waveform(dbl), element #2=w269:waveform(dbl))
                n126 = Match Pattern(string=w253, regular expression="15") -> (offset past match=w258:i32)  [unwired: 1 in, 3 out]
                n127 = Match Pattern(string=w253, regular expression="25") -> (offset past match=w255:i32)  [unwired: 1 in, 3 out]
                n128 = Unbundle By Name(w268) -> ("Y"=w263:dbl[])
                n129 = Unbundle By Name(w269) -> ("Y"=w262:dbl[])
                n130 = Less Than 0?(x=w258) -> (x < 0?=w259:bool)
                n131 = Less Than 0?(x=w255) -> (x < 0?=w256:bool)
                n132 = Not(x=w259) -> (.not. x?=w254:bool)
                n133 = Not(x=w256) -> (.not. x?=w251:bool)
                n134 = call <vilib>:"Std Deviation and Variance.vi"("X"=w263) -> ("mean"=→"Mean Qin_1":dbl, "standard deviation"=→"St. Deviation Qin_1":dbl, "variance"=→"Variance Qin_1":dbl)  [unwired: 1 in]
                n135 = call <vilib>:"Std Deviation and Variance.vi"("X"=w262) -> ("mean"=→"Mean Qin_2":dbl, "standard deviation"=→"St. Deviation Qin_2":dbl, "variance"=→"Variance Qin_2":dbl)  [unwired: 1 in]
                n136 = case shown="False" w254 {
                  tunnel: [w279 15] -> w252
                  tunnel: w251 -> [w280 _]
                  tunnel: [w278 0] -> w249
                  frame False {
                    n137 = case shown="False" w280 {
                      tunnel: [15 25] -> w279
                      tunnel: [25 0] -> w278
                      frame False {
                      }
                      frame True {
                      }
                    }
                  }
                  frame True {
                  }
                }
                n138 = Multiply(x=w250, y=w249) -> (x*y=w238:dbl)
                "Qin 2 (fCb)" <- w238
                n139 = Multiply(x=w252, y=w250) -> (x*y=w245:dbl)
                "Qin 1 (fCb)" <- w245
                n140 = Equal?(x=w238, y=4.5) -> (x = y?=w237:bool)
                n141 = Equal?(x=w245, y=4.5) -> (x = y?=w242:bool)
                n142 = Select(t=0.2 ("max"), s=w237, f=0.5) -> (s? t:f=w236:dbl)
                n143 = Select(t=0.2 ("max"), s=w242, f=0.5) -> (s? t:f=w243:dbl)
                n144 = call <vilib>:"General Histogram.vi"("X"=w263, "max"=w243, "min"=w248, "# bins"=w264) -> ("Histogram Graph"=w265:T6)  [unwired: 7 in, 4 out]
                n145 = call <vilib>:"General Histogram.vi"("X"=w262, "max"=w236, "min"=w248, "# bins"=w264) -> ("Histogram Graph"=w266:T6)  [unwired: 7 in, 4 out]
                n146 = property on="Cursor.Visible" class="Bool (strict)"("Visible"=w233) -> ()  [unwired: 2 in, 2 out]
                n147 = property on="Cursor.Visible 2" class="Bool (strict)"("Visible"=w233) -> ()  [unwired: 2 in, 2 out]
                n148 = property on="Time Difference" class="DigNum (strict)"("Visible"=w233) -> ()  [unwired: 2 in, 2 out]
                n149 = property on="Amplitude Difference" class="DigNum (strict)"("Visible"=w233) -> ()  [unwired: 2 in, 2 out]
                n150 = property on="Time Difference 2" class="DigNum (strict)"("Visible"=w233) -> ()  [unwired: 2 in, 2 out]
                n151 = property on="Amplitude Difference 2" class="DigNum (strict)"("Visible"=w233) -> ()  [unwired: 2 in, 2 out]
                n152 = Build Array(w265, w266) -> (→"Histogram":T2)
                n153 = property on="Linearity Graph" class="XYGraph (strict)"("Visible"=w235) -> ()  [unwired: 2 in, 2 out]
                n154 = property on="Pulser Waveform" class="WFGraph (strict)"("Visible"=w235) -> ()  [unwired: 2 in, 2 out]
                n155 = property on="Gain (mV/fCb)" class="DigNum (strict)"("Visible"=w235) -> ()  [unwired: 2 in, 2 out]
                n156 = property on="Simul. Graph" class="XYGraph (strict)"("Visible"=w235) -> ()  [unwired: 2 in, 2 out]
                n157 = property on="Load simulation Plot" class="Bool"("Visible"=w235) -> ()  [unwired: 2 in, 2 out]
                n158 = property on="Mean Qin_1" class="DigNum (strict)"("Visible"=w234) -> ()  [unwired: 2 in, 2 out]
                n159 = property on="St. Deviation Qin_1" class="DigNum (strict)"("Visible"=w234) -> ()  [unwired: 2 in, 2 out]
                n160 = property on="Variance Qin_1" class="DigNum (strict)"("Visible"=w234) -> ()  [unwired: 2 in, 2 out]
                n161 = property on="Mean Qin_2" class="DigNum (strict)"("Visible"=w234) -> ()  [unwired: 2 in, 2 out]
                n162 = property on="St. Deviation Qin_2" class="DigNum (strict)"("Visible"=w234) -> ()  [unwired: 2 in, 2 out]
                n163 = property on="Variance Qin_2" class="DigNum (strict)"("Visible"=w234) -> ()  [unwired: 2 in, 2 out]
                n164 = property on="Qin 1 (fCb)" class="DigNum (strict)"("Visible"=w234) -> ()  [unwired: 2 in, 2 out]
                n165 = property on="Qin 2 (fCb)" class="DigNum (strict)"("Visible"=w234) -> ()  [unwired: 2 in, 2 out]
                n166 = property on="Histogram" class="XYGraph (strict)"("Visible"=w234) -> ()  [unwired: 2 in, 2 out]
              }
            }
            n167 = case shown="Error" w166 {
              selector: w166 -> [w287 w297]
              tunnel: [w287 w296] -> w165
              frame No Error {
              }
              frame Error {
                # "Report error only within the TDMS error code range"
                n168 = Unbundle By Name(w297) -> ("code"=w293:i32, "source"=w298:string)
                n169 = In Range and Coerce(upper limit=-2500, x=w293, lower limit=-2550 ("upper limit")) -> (In Range?=w290:bool)  [unwired: 1 out]
                n170 = In Range and Coerce(upper limit=-68000, x=w293, lower limit=-68100) -> (In Range?=w289:bool)  [unwired: 1 out]
                n171 = Or(x=w290, y=w289) -> (x .or. y?=w288:bool)
                n172 = case shown="True" w288 {
                  tunnel: w298 -> [_ w304]
                  tunnel: w297 -> [w299 w303]
                  tunnel: [w299 w302] -> w296
                  tunnel: w293 -> [_ w300]
                  frame False {
                    # "Out of the range of TDMS\nerror code, we don't report\nthem."
                  }
                  frame True {
                    w301 = T7 4 items=["no dialog", "OK message", "continue or stop message", "OK message + warnings", "continue/stop + warnings"] ("type of dialog (OK msg:1)")
                    n173 = call <vilib>:"Simple Error Handler.vi"("error code (no error:0)"=w300, "error source (\" \")"=w304, "type of dialog (OK msg:1)"=w301, "error in (no error)"=w303) -> ("error out"=w302:errorcluster)  [unwired: 1 in, 4 out]
                  }
                }
              }
            }
            n174 = control-ref of="Raw data values"() -> (w180:refnum<vi>)
            n175 = property on="Raw data values" class="MCListbox (strict)"("ItemNames"=w181, "ColHdrString"=w175) -> ()  [unwired: 2 in, 2 out]
            n176 = property on="Waveform Graph" class="WFGraph (strict)"("XScale.NameLbl.Text"=w173, "YScale.NameLbl.Text"=w174) -> ()  [unwired: 2 in, 2 out]
            n177 = call <vilib>:"setListBoxColumnWidths.vi"("table data"=w181, "MCListbox Refnum"=w180) -> ()  [unwired: 1 out]
            n178 = property on="Waveform Graph" class="WFGraph (strict)"("XScale.LooseFit"=FALSE ("X Scale.Loose Fit")) -> ()  [unwired: 2 in, 2 out]
            n179 = call <vilib>:"Clear Errors.vi"("error in (no error)"=w165) -> ("error out"=w179:errorcluster)  [unwired: 1 in, 5 out]
          }
          event "Settings...": Value Change {
            n180 = event-data() -> ()  [unwired: 7 out]
            n181 = local read "File contents"() -> (w316:string)
            n182 = call <vilib>:"configureNumberOfValues.vi"("TDMS File Viewer Configuration"=w326) -> ("TDMS File Viewer Configuration Out"=w305:T4)  [unwired: 10 out]
            n183 = call <vilib>:"getNamesFromPath.vi"("error in (no error)"=w323, "tree path"=w316) -> ("error out"=w314:errorcluster, "channel"=w312:string, "group"=w313:string)  [unwired: 3 out]
            n184 = call <vilib>:"getChannelList.vi"("error in (no error)"=w314, "channel names"=w312, "group name"=w313, "tdms file"=w315) -> ("error out"=w311:errorcluster, "channel names out"=w308:string[], "group names out"=w309:string[], "tdms file out"=w310:refnum<k34>)
            n185 = call <vilib>:"loadAndFormatValues.vi"("error in (no error)"=w311, "configuration"=w305, "channel names"=w308, "group names"=w309, "tdms file"=w310) -> ("error out"=w324:errorcluster, "graph y names"=w318:string, "graph x names"=w317:string, "tdms file out"=w325:refnum<k34>, "waveform values"=w322:waveform(dbl)[], "table values"=w319:string[][], "table headers"=w321:string[])
            n186 = local read "Properties / Values / Graph"() -> (w306:T1)
            n187 = property on="Raw data values" class="MCListbox (strict)"("ItemNames"=w319, "ColHdrString"=w321) -> ()  [unwired: 2 in, 2 out]
            n188 = local write "Waveform Graph"(w322) -> ()
            n189 = control-ref of="Raw data values"() -> (w320:refnum<vi>)
            n190 = call <vilib>:"status.vi"("tab sheet"=w306, "TDMS File Viewer Configuration"=w305) -> ("status"=w307:string)  [unwired: 5 out]
            n191 = property on="Waveform Graph" class="WFGraph (strict)"("XScale.NameLbl.Text"=w317, "YScale.NameLbl.Text"=w318) -> ()  [unwired: 2 in, 2 out]
            n192 = local write "Status"(w307) -> ()
            n193 = call <vilib>:"setListBoxColumnWidths.vi"("table data"=w319, "MCListbox Refnum"=w320) -> ()  [unwired: 1 out]
          }
          event "Help": Value Change {
            n194 = event-data() -> ()  [unwired: 7 out]
            n195 = call <vilib>:"TDMSFileViewer_LaunchHelp.vi"("CHM or HLP filename (lvdialog.chm)"="lvdialog.chm", "HTML filename"="tdms_file_viewer_db.html") -> ()  [unwired: 1 in, 5 out]
          }
          event Panel Resize {
            n196 = event-data() -> ("NewBnds"=w336:T8)  [unwired: 1 out]
            n197 = call <vilib>:"panelResize.vi"("error in (no error)"=w334, "NewBnds"=w336, "control refs"=w335) -> ("error out"=w333:errorcluster)  [unwired: 4 in]
          }
          event Panel Close? {
            w338 = TRUE
            n198 = event-data() -> ()  [unwired: 5 out]
            n199 = event-data("Discard?"=w338) -> ()  [unwired: 1 in, 1 out]
          }
        }
        n200 = property on="Pulser Waveform" class="WFGraph (strict)"("Active Cursor"=u32 0, "Cursor.Visible"="Cursor.Visible", "Active Cursor"=u32 1, "Cursor.Visible"="Cursor.Visible") -> ("Cursor.Cursor X"=w85:dbl, "Cursor.Cursor Y"=w83:dbl, "Cursor.Cursor X"=w84:dbl, "Cursor.Cursor Y"=w82:dbl)  [unwired: 2 in, 2 out]
        n201 = property on="Simul. Graph" class="XYGraph (strict)"("Active Cursor"=u32 0, "Cursor.Visible"="Cursor.Visible 2", "Active Cursor"=u32 1, "Cursor.Visible"="Cursor.Visible 2") -> ("Cursor.Cursor X"=w76:dbl, "Cursor.Cursor Y"=w74:dbl, "Cursor.Cursor X"=w75:dbl, "Cursor.Cursor Y"=w73:dbl)  [unwired: 2 in, 2 out]
        n202 = Subtract(x=w85, y=w84) -> (x-y=→"Time Difference":dbl)
        n203 = Subtract(x=w83, y=w82) -> (x-y=→"Amplitude Difference":dbl)
        n204 = Subtract(x=w76, y=w75) -> (x-y=→"Time Difference 2":dbl)
        n205 = Subtract(x=w74, y=w73) -> (x-y=→"Amplitude Difference 2":dbl)
        n206 = case shown="True" "Load simulation Plot" {
          frame False {
          }
          frame True {
            n207 = call-poly <vilib>:"Read From Spreadsheet File.vi"("delimiter (\\t)"="," ("delimiter (\\t)"), "format (%.3f)"="%.;%.6f", "start of read offset (chars.:0)"=8) -> ("all rows"=w122:dbl[][])  [unwired: 4 in, 4 out]
            n208 = Index Array(array=w122, index (col) #1=0 ("index (row)"), index (col) #2=1 ("index (col)"), index (col) #3=2 ("index (col)"), index (col) #4=3 ("index (col)"), index (col) #5=4 ("index (col)"), index (col) #6=5 ("index (col)"), index (col) #7=6 ("index (col)"), index (col) #8=7 ("index (col)")) -> (element #1=w105:dbl[], element #2=w101:dbl[], element #3=w116:dbl[], element #4=w115:dbl[], element #5=w114:dbl[], element #6=w113:dbl[], element #7=w112:dbl[], element #8=w104:dbl[])  [unwired: 8 in]
            n209 = Bundle("all rows"=w105, "all rows"=w101) -> (w100:cluster{"all rows":dbl[], "all rows":dbl[]})  [unwired: 1 in]
            n210 = Bundle("all rows"=w105, "all rows"=w116) -> (w111:cluster{"all rows":dbl[], "all rows":dbl[]})  [unwired: 1 in]
            n211 = Bundle("all rows"=w105, "all rows"=w115) -> (w110:cluster{"all rows":dbl[], "all rows":dbl[]})  [unwired: 1 in]
            n212 = Bundle("all rows"=w105, "all rows"=w114) -> (w109:cluster{"all rows":dbl[], "all rows":dbl[]})  [unwired: 1 in]
            n213 = Bundle("all rows"=w105, "all rows"=w113) -> (w108:cluster{"all rows":dbl[], "all rows":dbl[]})  [unwired: 1 in]
            n214 = Bundle("all rows"=w105, "all rows"=w112) -> (w107:cluster{"all rows":dbl[], "all rows":dbl[]})  [unwired: 1 in]
            n215 = Bundle("all rows"=w105, "all rows"=w104) -> (w103:cluster{"all rows":dbl[], "all rows":dbl[]})  [unwired: 1 in]
            n216 = Build Array(w100, w111, w110, w109, w108, w107, w103) -> (→"Simul. Graph":cluster{"all rows":dbl[], "all rows":dbl[]}[])
          }
        }
      }
    }
    frame Error {
      n217 = call <vilib>:"Simple Error Handler.vi"("error in (no error)"=w342) -> ("error out"=w341:errorcluster)  [unwired: 1 in, 7 out]
    }
  }
  n218 = TDMS Close(8:w51, 11:w52) -> (0:w14:errorcluster)  [unwired: 1 out]
  n219 = case shown="True" w15 {
    tunnel: w14 -> [w344 w346]
    tunnel: [w344 w345] -> w13
    frame False {
    }
    frame True {
      n220 = invoke class="VI" method="FP.Close"(error in=w346) -> (error out=w345:errorcluster)  [unwired: 2 in, 2 out]
    }
  }
  "error out" <- w13
